vi "Shooter_Fire_2_1.vi"(8 "notThereIn":bool, 9 "Pot":dbl, 11 "Fire":bool) -> (0 "notThereOut":bool, 2 "PotOut":dbl, 3 "Power":dbl)   [LabVIEW 2013]
panel:
  out "InGear":bool
  in  "OutGearPos":dbl=2.1
  in  "InGearPos":dbl=1.5
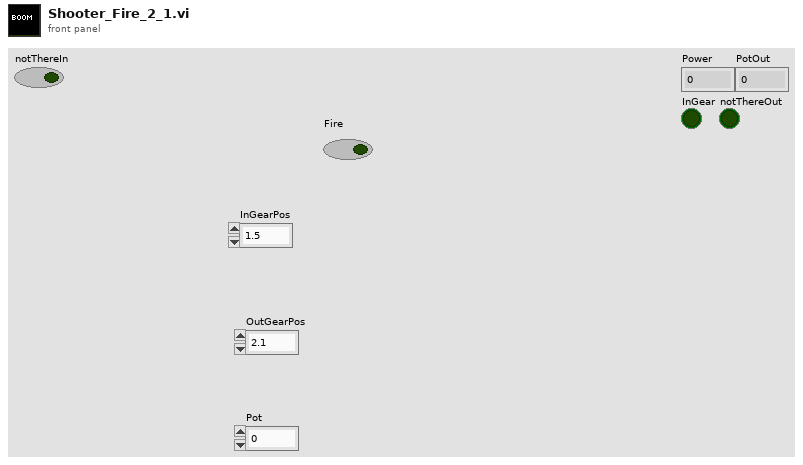
[diagram p1: front panel]
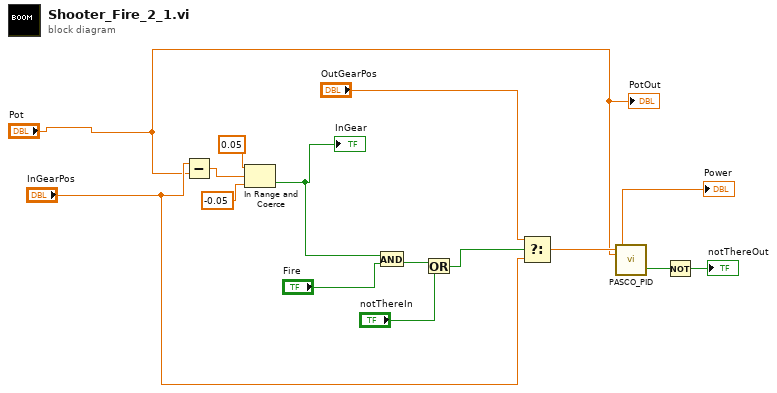
[diagram p0: block diagram]
diagram:
  n1 = Subtract(x="InGearPos", y="Pot") -> (x-y=w15:dbl)
  n2 = In Range and Coerce(upper limit=0.05, x=w15, lower limit=-0.05) -> (In Range?=w11:bool)  [unwired: 1 out]
  "InGear" <- w11
  n3 = And(x=w11, y="Fire") -> (x .and. y?=w1:bool)
  n4 = Or(x=w1, y="notThereIn") -> (x .or. y?=w9:bool)
  n5 = Select(t="OutGearPos", s=w9, f="InGearPos") -> (s? t:f=w8:dbl)
  n6 = call "PASCO_PID.vi"("Desired Rate"=w8, "Actual Rate"="Pot") -> ("Output"=→"Power":dbl, "IsThere"=w6:bool)  [unwired: 12 in]
  n7 = Not(x=w6) -> (.not. x?=→"notThereOut":bool)
  "PotOut" <- "Pot"
